vi "Generate File Footer.vi"(8 "error in (no error)":errorcluster, 11 "LUnit Test Vector in":refnum<class "LUnit Test Vector.lvclass">) -> (0 "error out":errorcluster, 2 "Header":string, 3 "LUnit Test Vector out":refnum<class "LUnit Test Vector.lvclass">)   [LabVIEW 2020, in "LUnit Test Vector.lvclass"]
uses:
  LUnit Test Vector.lvclass
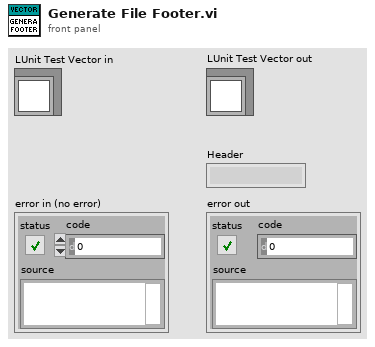
[diagram p1: front panel]
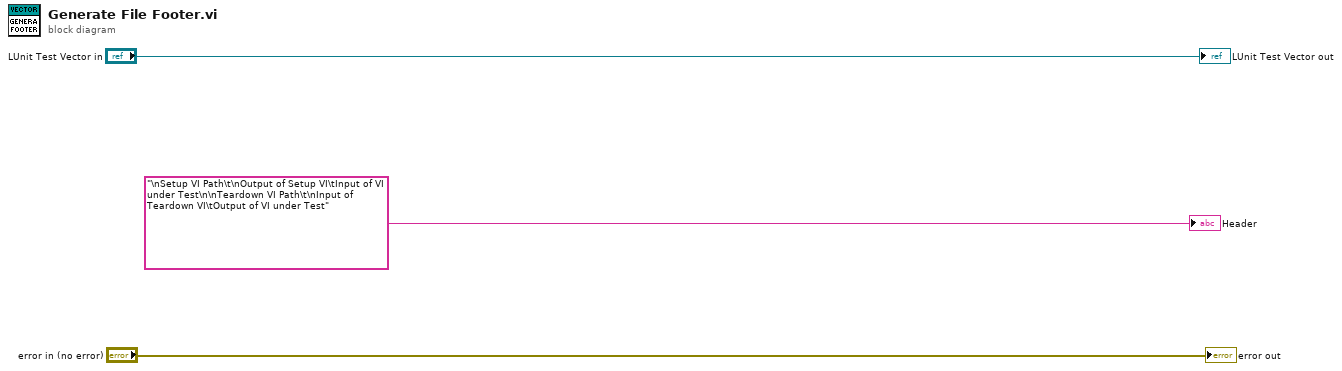
[diagram p0: block diagram]
diagram:
  "Header" <- "\nSetup VI Path\t\nOutput of Setup VI\tInput of VI under Test\n\nTeardown VI Path\t\nInput of Teardown VI\tOutput of VI under Test"
  "error out" <- "error in (no error)"
  "LUnit Test Vector out" <- "LUnit Test Vector in"
